vi "potenciometros.vi"() -> ()   [LabVIEW 2025]
uses:
  <vilib>/Instr/_visa.llb/VISA Configure Serial Port (Instr).vi
panel:
  out "Buffer":string
  in  "Puerto COM:":refnum<visa-resource-name>
  in  "stop":bool
  out "Temperatura":dbl(slide) scale=0.0..150.0
  out "Gasolina":dbl(slide) scale=0.0..100.0
  out "Bateria":dbl(knob) scale=0.0..12.0
  out "Velocidad":dbl(knob) scale=0.0..220.0
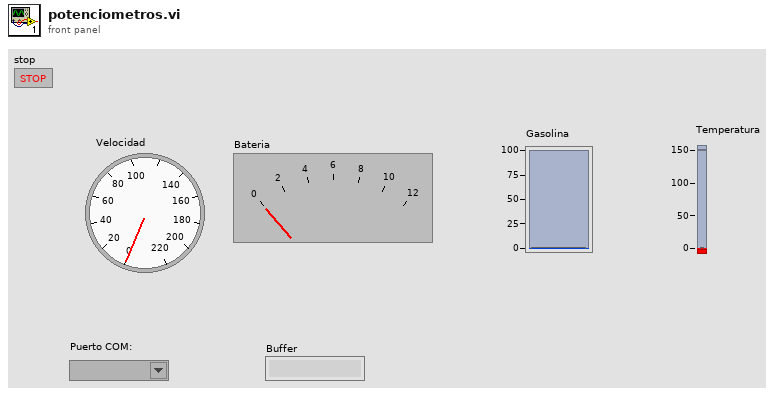
[diagram p1: front panel]
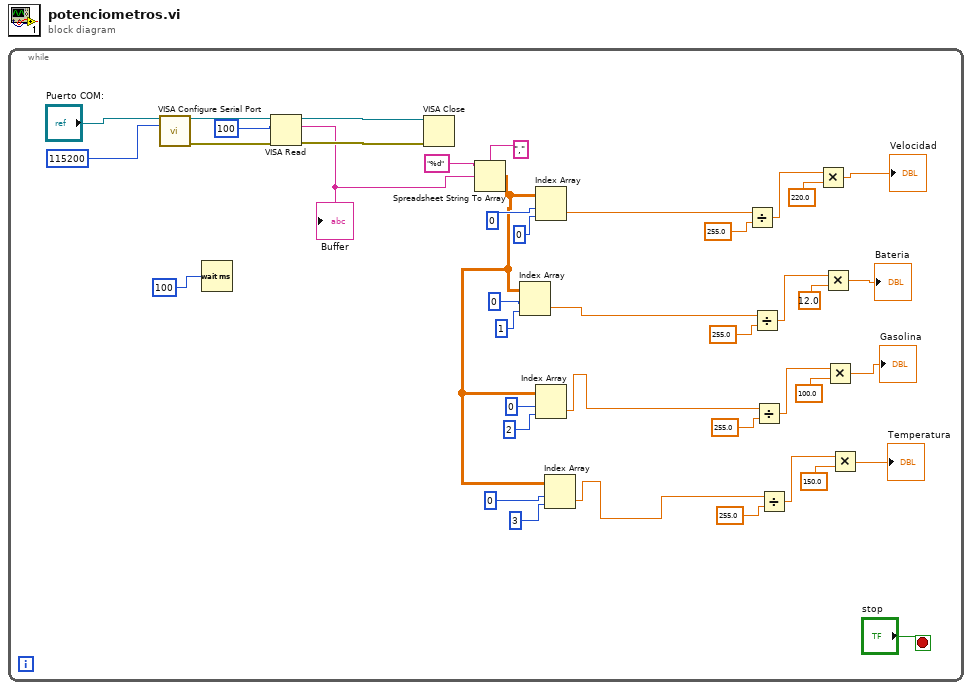
[diagram p0: block diagram]
diagram:
  n1 = while {
    stop <- "stop" stop-if-true
    n2 = call-poly "VISA Configure Serial Port"("VISA resource name"="Puerto COM:", "baud rate (9600)"=u32 115200) -> ("VISA resource name out"=w37:refnum<visa-resource-name>, "error out"=w38:errorcluster)  [unwired: 12 in]
    n3 = Wait (ms)(milliseconds to wait=u32 100) -> ()  [unwired: 1 out]
    n4 = VISA Read(VISA resource name=w37, byte count=u32 100, error in (no error)=w38) -> (VISA resource name out=w34:refnum<visa-resource-name>, read buffer=w28:string, error out=w35:errorcluster)  [unwired: 1 out]
    "Buffer" <- w28
    n5 = VISA Close(VISA resource name=w34, error in (no error)=w35) -> ()  [unwired: 1 out]
    n6 = Spreadsheet String To Array(delimiter (Tab)=",", format string="%d", spreadsheet string=w28) -> (array=w8:dbl[][])  [unwired: 1 in]
    n7 = Index Array(array=w8, index (row)=0, index (col)=1) -> (element=w17:dbl)
    n8 = Index Array(array=w8, index (row)=0, index (col)=0) -> (element=w23:dbl)
    n9 = Index Array(array=w8, index (row)=0, index (col)=2) -> (element=w10:dbl)
    n10 = Index Array(array=w8, index (row)=0, index (col)=3) -> (element=w2:dbl)
    n11 = Divide(x=w23, y=255.0) -> (x/y=w31:dbl)
    n12 = Divide(x=w17, y=255.0) -> (x/y=w18:dbl)
    n13 = Divide(x=w10, y=255.0) -> (x/y=w11:dbl)
    n14 = Divide(x=w2, y=255.0) -> (x/y=w3:dbl)
    n15 = Multiply(x=w31, y=220.0) -> (x*y=→"Velocidad":dbl)
    n16 = Multiply(x=w18, y=12.0) -> (x*y=→"Bateria":dbl)
    n17 = Multiply(x=w11, y=100.0) -> (x*y=→"Gasolina":dbl)
    n18 = Multiply(x=w3, y=150.0) -> (x*y=→"Temperatura":dbl)
  }
